vi "Video File Close.vi"(8 "error in (no error)":errorcluster, 11 "Video File in":refnum<class "Video File.lvclass">) -> (0 "error out":errorcluster, 3 "Video File out":refnum<class "Video File.lvclass">)   [LabVIEW 2018, in "Video File.lvclass"]
uses:
  Video File.lvclass
  Video File.lvclass/Video File.ctl
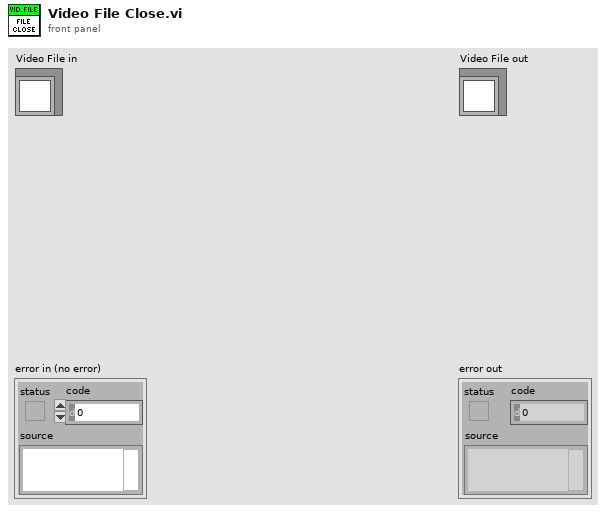
[diagram p1: front panel]
types:
  T1 = typedef "IMAQ AVI2 Refnum.ctl" = refnum<k20>
  T2 = typedef "IMAQ Image.ctl" = refnum<image>
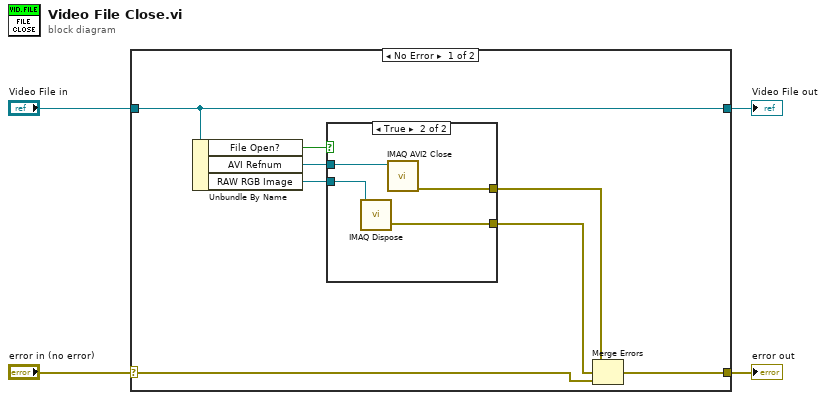
[diagram p0: block diagram]
diagram:
  n1 = case shown="No Error" "error in (no error)" {
    selector: "error in (no error)" -> [w6 w18]
    tunnel: [w9 w18] -> w3
    tunnel: [w12 w17] -> w1
    tunnel: "Video File in" -> [w12 w17]
    frame No Error {
      n2 = Unbundle By Name(w12) -> ("File Open?"=w5:bool, "AVI Refnum"=w11:T1, "RAW RGB Image"=w10:T2)
      n3 = case shown="True" w5 {
        tunnel: w11 -> [_ w16]
        tunnel: w10 -> [_ w15]
        tunnel: [_ w14] -> w8
        tunnel: [_ w13] -> w7
        frame False {
        }
        frame True {
          n4 = call "IMAQ Dispose"("Image"=w15) -> ("error out"=w13:errorcluster)  [unwired: 2 in, 3 out]
          n5 = call "IMAQ AVI2 Close"("AVI Refnum"=w16) -> ("error out"=w14:errorcluster)  [unwired: 1 in, 9 out]
        }
      }
      n6 = Merge Errors(w8, w7, w6) -> (w9:errorcluster)
    }
    frame Error {
    }
  }
  "error out" <- w3
  "Video File out" <- w1
